vi "AttributeGuide.vi"() -> (15 "Preview":string, 16 "Canceled":bool)   [LabVIEW 2012, in "ClassNode.lvclass"]
uses:
  <resource>/Framework/Providers/Open_GDS/UML/ClassNode_class/ClassNode.lvclass
  <resource>/Framework/Providers/Open_GDS/ClassProviders/Common/CommonVIs/CommonVIs_AttributeDataType.ctl
  <resource>/Framework/Providers/Open_GDS/UML/ContextHelp/ContextHelp_HelpTexts.ctl
panel:
  in  "Help":bool
  in  "RefName":string
  in  "Cancel":bool
  in  "OK":bool
  in  "Array?":u16(ring) items=["No", "1D", "2D", "3D"]
  in  "AttributeName":string
  in  "Data Type":T1
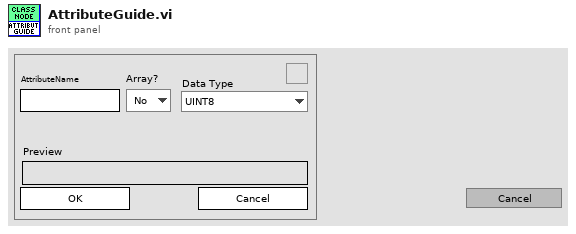
[diagram p1: front panel]
types:
  T1 = typedef "CommonVIs_AttributeDataType.ctl" = enum16{"UINT8", "INT8", "UINT16", "INT16", "UINT32", "INT32", "UINT64", "INT64", "SGL", "DBL", "EXT", "CSG", "CDB", "CXT", "TimeStamp", "STRING", "PATH", "BOOL", "ENUM", "RefNum", "VIRefNum", "LabVIEW Class", "Cluster", "Variant", "TypeDef", "Waveform", "LabVIEW Object", "Other", "void"}
  T2 = typedef "ContextHelp_HelpTexts.ctl" = enum16{"None(Hide)", "Default", "Help", "Welcome", "GettingStarted", "ClassDiagram_Help", "SequenceDiagram_Help", "UseCaseDiagram_Help", "BSelect", "BClass", "BInterface", "BPackage", "BNote", "BDependency", "BInheritance", "BInterfaceImplementation", "BAssociation", "BAggregation", "BCompAggregation", "BNoteConnector", "BObject", "BActionBar", "BCall", "BSystem", "BActor", "BUseCase", "BGeneralization", "BIncludes", "BExtends", "BUseCaseDiagramAssociation", "ClassRelationshipEdge editDialog_Bent Style", "ClassRelationshipEdge editDialog_RelationType", "ClassRelationshipEdge editDialog_Reverse association", "ClassRelationshipEdge editDialog_Start label", "ClassRelationshipEdge editDialog_Middle label", "ClassRelationshipEdge editDialog_End label", "UMLEditor reversedEngineering_Pathes", "ReversedEngineering StateReverseDialog_Help", "ReversedEngineering StateQueuedSettings_Help", "UMLEditor reversedEngineering_AddTopVIs", "UMLEditor reversedEngineering_AddClasses", "UMLEditor reversedEngineering_AddDirs", "UMLEditor reversedEngineering_Recursively", "UMLEditor reversedEngineering_Remove", "UMLEditor reversedEngineering_ClearList", "UMLEditor reversedEngineering_HideSubAss", "UMLEditor reversedEngineering_CreateTypes", "UMLEditor reversedEngineering_OnlyInheritance", "UMLEditor reversedEngineering_CreateApplication", "UMLEditor reversedEngineering_OK", "UMLEditor reversedEngineering_Cancel", "UMLEditor reversedEngineering_Help", "UMLEditor createWizardScriptFile_ScriptfilePath", "UMLEditor createWizardScriptFile_ClassPath", "UMLEditor createWizardScriptFile_Use", "UMLEditor createWizardScriptFile_PrivateDirName", "UMLEditor createWizardScriptFile_DirAppend", "UMLEditor createWizardScriptFile_Separator Character", "UMLEditor createWizardScriptFile_OK", "UMLEditor createWizardScriptFile_Cancel", "UMLEditor createWizardScriptFile_Help", "ClassNode editDialog_Class Name", "InterfaceNode editDialog_Class Name", "ClassNode editDialog_Attribute", "ClassNode editDialog_Methods", "InterfaceNode editDialog_Methods", "ClassNode editDialog_connection", "InterfaceNode editDialog_connection", "ClassNode editDialog_StereoType", "ClassNode editDialog_ShowAttrib", "ClassNode editDialog_ShowMethods", "ClassNode editDialog_ClassPath", "ClassNode editDialog_AddAttribute", "ClassNode editDialog_AddMethod", "InterfaceNode editDialog_AddMethod", "ClassNode AttributeGuide_AttributeName", "ClassNode AttributeGuide_Array?", "ClassNode AttributeGuide_Data Type", "ClassNode AttributeGuide_RefName", "ClassNode AttributeGuide_Preview", "ClassNode AttributeGuide_OK", "ClassNode AttributeGuide_Cancel", "ClassNode MethodGuide_Visibility", "ClassNode MethodGuide_Method Name", "ClassNode MethodGuide_Preview", "ClassNode MethodGuide_OK", "ClassNode MethodGuide_Cancel", "CallNode EditCallProperties_AllButtons", "ObjectNode EditObjectlProperties_AllButtons", "ActorNode EditActorProperties_AllButtons", "UseCaseRelationshipNode EditUseCaselProperties_AllButtons", "UseCaseNode EditUseCaselProperties_AllButtons", "SystemNode EditSystemProperties_AllButtons", "ReversedEngineering UpdateAttributes_AllButtons", "StateNode editDialog_AllButtons", "StateTransition editDialog_AllButtons", "ArrangeNodes Main_Picture", "ArrangeNodes Main_Zoom", "ArrangeNodes Main_Auto Zoom", "ArrangeNodes Main_shorten", "ArrangeNodes Main_Min Length", "ArrangeNodes Main_Max Length", "ArrangeNodes Main_increase", "ArrangeNodes Main_decrease", "ArrangeNodes Main_Shake", "ArrangeNodes Main", "BState", "BInitialState", "BFinalState", "BStateTransition", "StateDiagram_Help", "StateDiagram_PropertiesAllButtons", "ReversedEngineering StateReverseDialog_ClearStates", "ReversedEngineering StateReverseDialog_UseQueuedStateMachines", "ReversedEngineering StateReverseDialog_QueuedSettings", "ReversedEngineering StateReverseDialog_SearchForVIs", "ReversedEngineering StateReverseDialog_SearchCriteria", "OptionsDialog_ClassBasePath", "OptionsDialog_VIPath", "OptionsDialog_ApplicationPath", "OptionsDialog_WizDir", "OptionsDialog_IniFilePath", "OptionsDialog_DefineColors", "OptionsDialog_Help", "OptionsDialog_CreateTypes", "ClassRelationshipEdge editDialog_SplitWire"}
  T3 = typedef "ContextHelp_ShowType.ctl" = cluster{"Header":string, "Picture":picture, "Text":string}
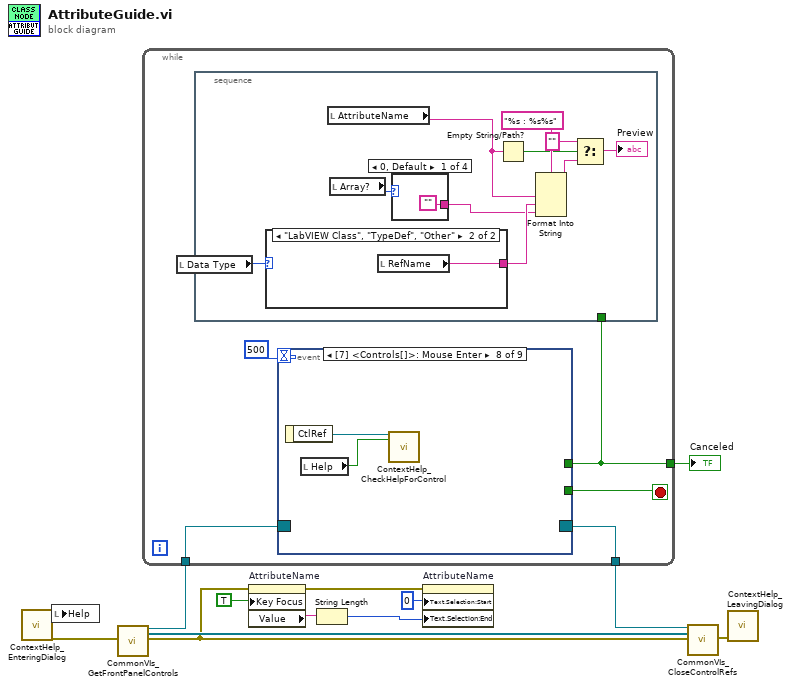
[diagram p0: block diagram]
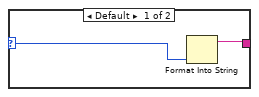
[diagram p2: hidden frame]
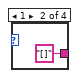
[diagram p3: hidden frame]
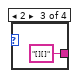
[diagram p4: hidden frame]
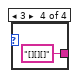
[diagram p5: hidden frame]
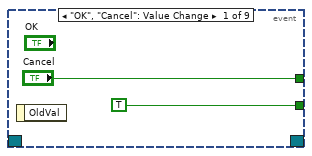
[diagram p6: hidden frame]
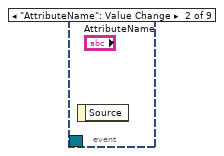
[diagram p7: hidden frame]
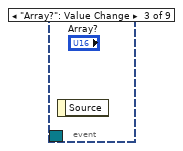
[diagram p8: hidden frame]
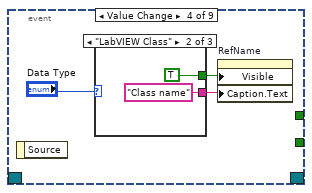
[diagram p9: hidden frame]
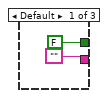
[diagram p10: hidden frame]
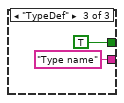
[diagram p11: hidden frame]
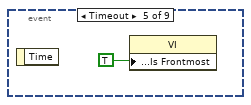
[diagram p12: hidden frame]
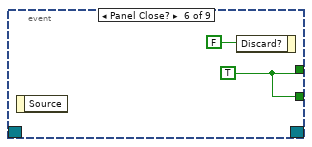
[diagram p13: hidden frame]
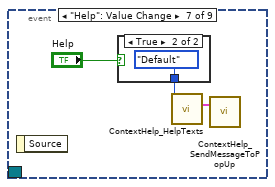
[diagram p14: hidden frame]
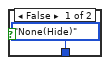
[diagram p15: hidden frame]
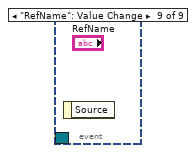
[diagram p16: hidden frame]
diagram:
  n1 = call <resource>:"ContextHelp_EnteringDialog.vi"() -> ("HelpStatus"=w12:bool, "error out"=w10:errorcluster)  [unwired: 3 in, 15 out]
  n2 = local write "Help"(w12) -> ()
  n3 = call <resource>:"CommonVIs_GetFrontPanelControls.vi"("error in (no error)"=w10) -> ("Event Registration Refnum"=w8:refnum<event-registration>, "ControlRefs"=w11:refnum<vi>[], "error out"=w5:errorcluster)  [unwired: 1 in, 15 out]
  n4 = while {
    tunnel: [w14] -> w13
    tunnel: w8 -> [w17]
    tunnel: [w16] -> w7
    stop <- w18 stop-if-true
    n5 = event shown="[7] <Controls[]>: Mouse Enter" {
      selector: w17 -> [_ _ _ _ _ _ _ _ _]
      dyn-events: [_ _ _ _ _ _ _ _ _] -> w16
      timeout: 500 -> [_ _ _ _ _ _ _ _ _]
      tunnel: ["Cancel" _ _ _ _ w48 _ _ _] -> w14
      tunnel: [TRUE _ _ _ _ w48 _ _ _] -> w18
      event "OK", "Cancel": Value Change {
        n6 = event-data() -> ()  [unwired: 2 out]
      }
      event "AttributeName": Value Change {
        n7 = event-data() -> ()  [unwired: 2 out]
      }
      event "Array?": Value Change {
        n8 = event-data() -> ()  [unwired: 2 out]
      }
      event Value Change {
        n9 = event-data() -> ()  [unwired: 2 out]
        n10 = case shown="\"LabVIEW Class\"" "Data Type" {
          tunnel: ["" "Class name" "Type name"] -> w38
          tunnel: [FALSE TRUE TRUE] -> w39
          frame Default {
          }
          frame "LabVIEW Class" {
          }
          frame "TypeDef" {
          }
        }
        n11 = property on="RefName" class="Str"("Visible"=w39, "Caption.Text"=w38) -> ()  [unwired: 2 in, 2 out]
      }
      event Timeout {
        n12 = event-data() -> ()  [unwired: 2 out]
        n13 = property class="VI"("Front Panel Window:Is Frontmost"=TRUE) -> ()  [unwired: 2 in, 2 out]
      }
      event Panel Close? {
        w48 = TRUE ("Discard?")
        n14 = event-data() -> ()  [unwired: 2 out]
        n15 = event-data("Discard?"=FALSE) -> ()  [unwired: 1 in, 1 out]
      }
      event "Help": Value Change {
        n16 = event-data() -> ()  [unwired: 2 out]
        n17 = case shown="True" "Help" {
          tunnel: [ContextHelp_HelpTexts."None(Hide)" ("HelpText") ContextHelp_HelpTexts."Default" ("HelpText")] -> w51
          frame False {
          }
          frame True {
          }
        }
        n18 = call <resource>:"ContextHelp_HelpTexts.vi"("HelpText (enum or string)"=w51) -> ("HelpOut"=w50:T3)  [unwired: 18 out]
        n19 = call <resource>:"ContextHelp_SendMessageToPopUp.vi"("PopUpMessage"=w50) -> ()  [unwired: 2 in, 17 out]
      }
      event Mouse Enter {
        n20 = event-data() -> ("CtlRef"=w56:refnum<vi>)  [unwired: 1 out]
        n21 = local read "Help"() -> (w55:bool)
        n22 = call <resource>:"ContextHelp_CheckHelpForControl.vi"("Ctl Refnum"=w56, "Help"=w55) -> ()  [unwired: 1 in, 17 out]
      }
      event "RefName": Value Change {
        n23 = event-data() -> ()  [unwired: 2 out]
      }
    }
    n24 = stacked-sequence {
      tunnel: w14 -> [_]
      frame #0 {
        n25 = local read "Data Type"() -> (w26:T1)
        n26 = case shown="\"LabVIEW Class\", \"TypeDef\", \"Other\"" w26 {
          selector: w26 -> [w30 _]
          tunnel: [w29 w31] -> w21
          frame Default {
            n27 = Format Into String(w30) -> (resulting string=w29:string)  [unwired: 3 in, 1 out]
          }
          frame "LabVIEW Class", "TypeDef", "Other" {
            n28 = local read "RefName"() -> (w31:string)
          }
        }
        n29 = local read "AttributeName"() -> (w25:string)
        n30 = local read "Array?"() -> (w27:u16)
        n31 = case shown="0, Default" w27 {
          tunnel: ["" "[]" "[][]" "[][][]"] -> w20
          frame 0, Default {
          }
          frame 1 {
          }
          frame 2 {
          }
          frame 3 {
          }
        }
        n32 = Empty String/Path?(string/path=w25) -> (empty?=w24:bool)
        n33 = Format Into String(format string="%s : %s%s", w25, w21, w20) -> (resulting string=w23:string)  [unwired: 2 in, 1 out]
        n34 = Select(t="", s=w24, f=w23) -> (s? t:f=→"Preview":string)
      }
    }
  }
  "Canceled" <- w13
  n35 = property on="AttributeName" class="Str"(error in=w5, "Key Focus"=TRUE) -> (error out=w3:errorcluster, "Value"=w4:string)  [unwired: 1 in, 1 out]
  n36 = String Length(string=w4) -> (length=w1:i32)
  n37 = property on="AttributeName" class="Str"(error in=w3, "Text.Selection:Start"=u32 0, "Text.Selection:End"=w1) -> ()  [unwired: 1 in, 2 out]
  n38 = call <resource>:"CommonVIs_CloseControlRefs.vi"("Event Registration Refnum"=w7, "ControlRefs"=w11, "error in (no error)"=w5) -> ("error out"=w9:errorcluster)  [unwired: 16 out]
  n39 = call <resource>:"ContextHelp_LeavingDialog.vi"("error in (no error)"=w9) -> ()  [unwired: 2 in, 17 out]
